vi "receive_02trigger.vi"() -> ()   [LabVIEW 2015]
uses:
  <instrlib>/niUSRP/niUSRP Fetch Rx Data (CDB Cluster).vi
panel:
  out "Filename Out":path
  out "Saving Data":bool
  out "Triggered Signal":dynamicdata(graph)
  out "Data Available":bool
  in  "active antenna":string="RX2"
  in  "Channels":string(combo)="0"
  out "Waveform Magnitude":cluster{"t0":dbl, "dt":dbl, "Y":dbl[]}(graph)
  in  "Stop":bool
  out "coerced gain":dbl format="%#_6f"
  out "coerced carrier frequency":dbl=100000.0 format="%#_6p"
  out "coerced IQ rate":dbl=100000.0 format="%#_6p"
  in  "gain":dbl format="%#_6f"
  in  "carrier frequency":dbl=920000000.0 format="%#_6p"
  in  "IQ rate":dbl=2000000.0 format="%#_6p"
  in  "number of samples":i64=2000000
  in  "timeout":dbl=10.0
  out "error out":errorcluster
  in  "device names":refnum<k15>="192.168.10.14"
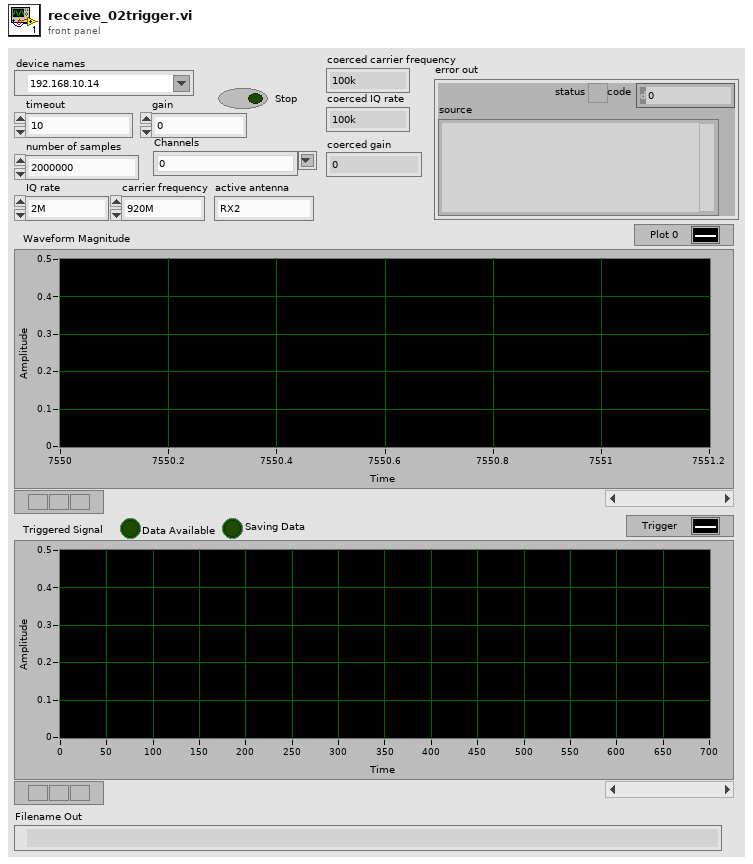
[diagram p1: front panel]
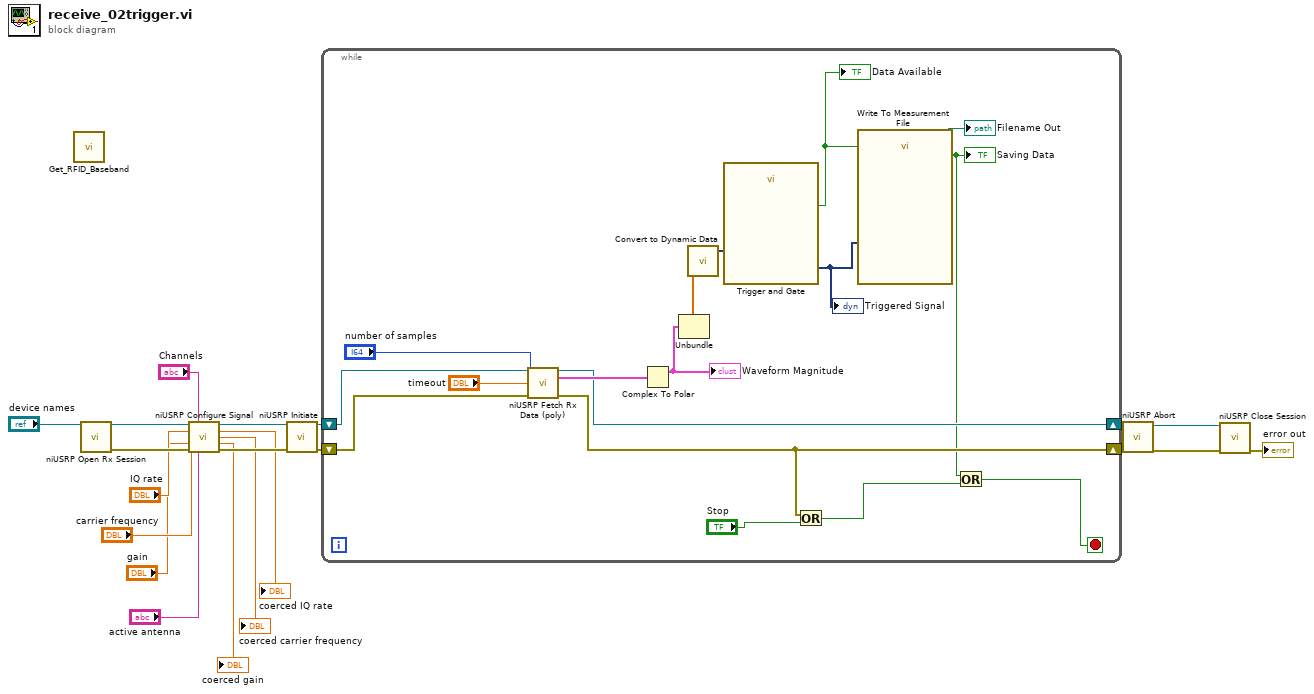
[diagram p0: block diagram]
diagram:
  n1 = call "Get_RFID_Baseband.vi"() -> ()  [unwired: 14 in, 2 out]
  n2 = call <instrlib>:"niUSRP Open Rx Session.vi"("device names"="device names") -> ("session handle out"=w19:refnum<k15>, "error out"=w18:errorcluster)  [unwired: 13 in]
  n3 = call <instrlib>:"niUSRP Configure Signal.vi"("session handle"=w19, "channel list"="Channels", "IQ rate"="IQ rate", "carrier frequency"="carrier frequency", "gain"="gain", "error in (no error)"=w18, "active antenna"="active antenna") -> ("session handle out"=w17:refnum<k15>, "coerced IQ rate"=→"coerced IQ rate":dbl, "coerced carrier frequency"=→"coerced carrier frequency":dbl, "coerced gain"=→"coerced gain":dbl, "error out"=w16:errorcluster)  [unwired: 4 in]
  n4 = call <instrlib>:"niUSRP Initiate.vi"("session handle"=w17, "error in (no error)"=w16) -> ("session handle out"=w15:refnum<k15>, "error out"=w14:errorcluster)  [unwired: 12 in]
  n5 = while {
    shift-right: [w33] -> w13
    shift-left: w15 -> [w32]
    shift-right: [w30] -> w12
    shift-left: w14 -> [w31]
    stop <- w22 stop-if-true
    n6 = call-poly <instrlib>:"niUSRP Fetch Rx Data (poly).vi"("session handle"=w32, "number of samples"="number of samples", "timeout"="timeout", "error in (no error)"=w31) -> ("session handle out"=w33:refnum<k15>, "data"=w34:cluster{"t0":dbl, "dt":dbl, "Y":cdb[]}, "error out"=w30:errorcluster)  [unwired: 8 in, 1 out]
    n7 = Complex To Polar(r * e^(i*theta)=w34) -> (r=w29:cluster{"t0":dbl, "dt":dbl, "Y":dbl[]})  [unwired: 1 out]
    "Waveform Magnitude" <- w29
    n8 = Unbundle(w29) -> ("Y"=w28:dbl[])  [unwired: 2 out]
    n9 = call "Convert to Dynamic Data"("Array"=w28) -> ("Dynamic Data Type"=w27:dynamicdata)  [unwired: 3 in]
    n10 = call "Trigger and Gate"("Signals"=w27) -> ("Triggered Signals"=w25:dynamicdata, "Data Available"=w26:bool)  [unwired: 7 in, 2 out]
    "Data Available" <- w26
    "Triggered Signal" <- w25
    n11 = Or(x=w30, y="Stop") -> (x .or. y?=w23:bool)
    n12 = call "Write To Measurement File"("Signals"=w25, "Enable"=w26) -> ("Filename Out"=→"Filename Out":path, "Saving Data"=w21:bool)  [unwired: 15 in, 1 out]
    "Saving Data" <- w21
    n13 = Or(x=w21, y=w23) -> (x .or. y?=w22:bool)
  }
  n14 = call <instrlib>:"niUSRP Abort.vi"("session handle"=w13, "error in (no error)"=w12) -> ("session handle out"=w11:refnum<k15>, "error out"=w10:errorcluster)  [unwired: 12 in]
  n15 = call <instrlib>:"niUSRP Close Session.vi"("session handle"=w11, "error in (no error)"=w10) -> ("error out"=→"error out":errorcluster)  [unwired: 13 in]
